vi "CTRE_Phoenix_MotorController_GetClosedLoopData.vi"(0 "PhoenixMotorControlDevRef":T1={"DeviceStatus"={"status"=FALSE, "code"=0, "source"=""}, "Type"=enum."PWM", "PWM"={"PWM Channel"=enum."Invalid", "DeadBand"={"Name"="", "maxPositivePwm"=0, "minPositivePwm"=0, "centerPwm"=0, "maxNegativePwm"=0, "minNegativePwm"=0, "angularRange"=0}}, "CAN"={"Device Number"=0, "SetOutput VI Ref"=variant(enum8{"Percent VBus", "Current", "Speed", "Position", "Voltage"} enum."Percent VBus"), "GetOutput VI Ref"=variant(refnum<k1> refnum), "Enable VI Ref"=variant(dbl 12.0), "Disable VI Ref"=variant(enum8{"Percent VBus", "Speed", "Position", "Slave", "Unchanged / Invalid", "Voltage Compensation", "Current", "Motion Profile"} enum."Percent VBus"), "Data"=variant}, "Invert"=FALSE, "DIO PWM"={"PWM \"Enable\" Channel"=enum."Invalid", "DIOChannel"=enum."Invalid", "PWM Rate"=0.0}}, 5 "pidLoopIdx":i32, 11 "error in":errorcluster) -> (3 "Closed-loop Target":i32, 4 "PhoenixMotorControlDevRef":T1={"DeviceStatus"={"status"=FALSE, "code"=0, "source"=""}, "Type"=enum."PWM", "PWM"={"PWM Channel"=enum."Invalid", "DeadBand"={"Name"="", "maxPositivePwm"=0, "minPositivePwm"=0, "centerPwm"=0, "maxNegativePwm"=0, "minNegativePwm"=0, "angularRange"=0}}, "CAN"={"Device Number"=0, "SetOutput VI Ref"=variant(enum8{"Percent VBus", "Current", "Speed", "Position", "Voltage"} enum."Percent VBus"), "GetOutput VI Ref"=variant(refnum<k1> refnum), "Enable VI Ref"=variant(dbl 12.0), "Disable VI Ref"=variant(enum8{"Percent VBus", "Speed", "Position", "Slave", "Unchanged / Invalid", "Voltage Compensation", "Current", "Motion Profile"} enum."Percent VBus"), "Data"=variant}, "Invert"=FALSE, "DIO PWM"={"PWM \"Enable\" Channel"=enum."Invalid", "DIOChannel"=enum."Invalid", "PWM Rate"=0.0}}, 6 "Closed-loop Error":i32, 8 "Error Derivative":dbl, 10 "Integral Accumulator":dbl, 15 "error out":errorcluster)   [LabVIEW 2017]
doc: "<b> pidLoopIdx </b> The selected PID object to retrieve information from. Select 0 for primary, 1 for secondary (cascaded) PID loop.\nReturns the closed-loop data of the motor controller, including:\n\nClosed-loop Target\nClosed-loop Error\nError Derivative\nIntegral Accumulator"
uses:
  <vilib>/Rock Robotics/WPI/MotorControl/WPI_MotorControlDeviceRef.ctl
  <vilib>/Rock Robotics/WPI/MotorControl/WPI_MotorControlType.ctl
  <vilib>/Rock Robotics/SystemInterfaces/DIO/FPGA_DIOPWMChannel.ctl
  <vilib>/Rock Robotics/WPI/PWM/WPI_PWMDeadband.ctl
  <vilib>/Rock Robotics/SystemInterfaces/DIO/FPGA_DIOChannel.ctl
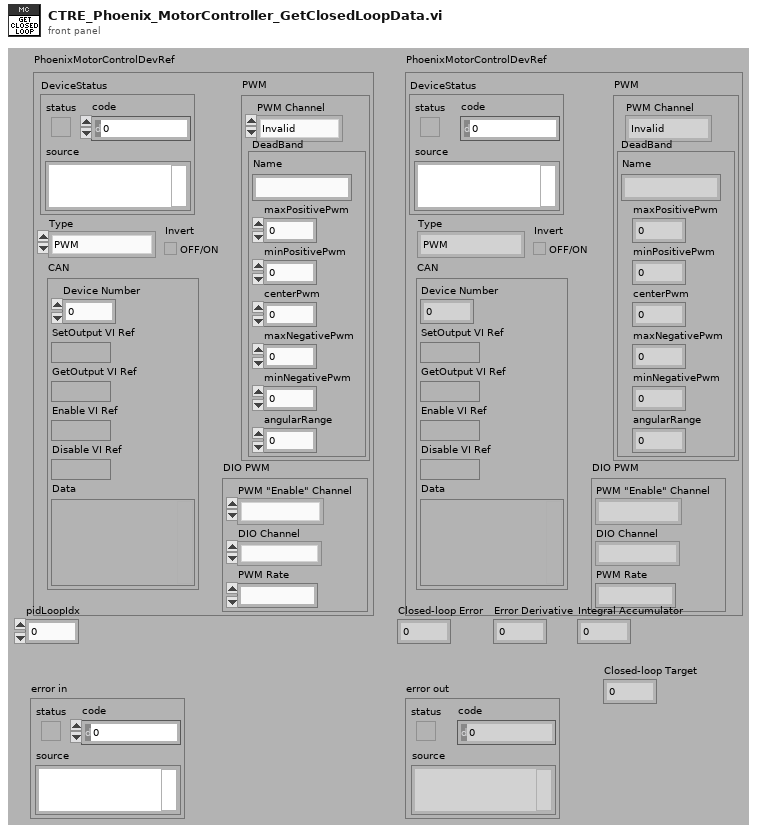
[diagram p1: front panel]
types:
  T1 = typedef "WPI_MotorControlDeviceRef.ctl" = cluster{"DeviceStatus":errorcluster, "Type":T2, "PWM":cluster{"PWM Channel":T3, "DeadBand":T4}, "CAN":cluster{"Device Number":u8, "SetOutput VI Ref":variant, "GetOutput VI Ref":variant, "Enable VI Ref":variant, "Disable VI Ref":variant, "Data":variant}, "Invert":bool, "DIO PWM":cluster{"PWM \"Enable\" Channel":T3, "DIOChannel":T5, "PWM Rate":dbl}}
  T2 = typedef "WPI_MotorControlType.ctl" = enum16{"PWM", "CAN", "DIO PWM"}
  T3 = typedef "FPGA_DIOPWMChannel.ctl" = enum8{"PWM 0", "PWM 1", "PWM 2", "PWM 3", "PWM 4", "PWM 5", "PWM 6", "PWM 7", "PWM 8", "PWM 9", "PWM MXP 0", "PWM MXP 1", "PWM MXP 2", "PWM MXP 3", "PWM MXP 4", "PWM MXP 5", "PWM MXP 6", "PWM MXP 7", "PWM MXP 8", "PWM MXP 9", "Invalid"}
  T4 = typedef "WPI_PWMDeadband.ctl" = cluster{"Name":string, "maxPositivePwm":i32, "minPositivePwm":i32, "centerPwm":i32, "maxNegativePwm":i32, "minNegativePwm":i32, "angularRange":u16}
  T5 = typedef "FPGA_DIOChannel.ctl" = enum8{"DIO 0", "DIO 1", "DIO 2", "DIO 3", "DIO 4", "DIO 5", "DIO 6", "DIO 7", "DIO 8", "DIO 9", "DIO MXP 0", "DIO MXP 1", "DIO MXP 2", "DIO MXP 3", "DIO MXP 4", "DIO MXP 5", "DIO MXP 6", "DIO MXP 7", "DIO MXP 8", "DIO MXP 9", "DIO MXP 10", "DIO MXP 11", "DIO MXP 12", "DIO MXP 13", "DIO MXP 14", "DIO MXP 15", "SPI Port CS1", "SPI Port CS2", "SPI Port CS3", "SPI Port MISO", "SPI Port MOSI", "Invalid"}
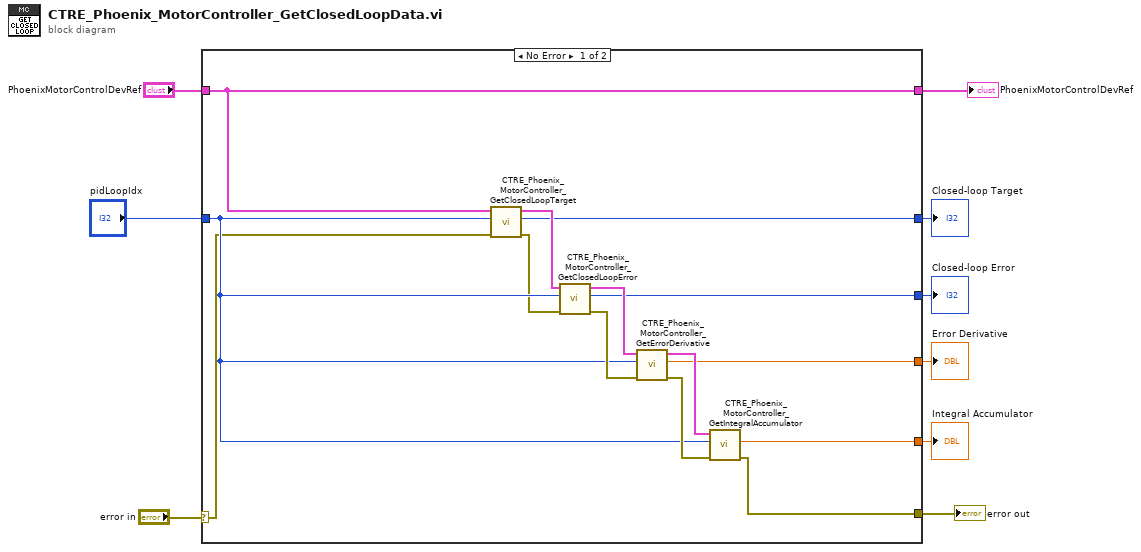
[diagram p0: block diagram]
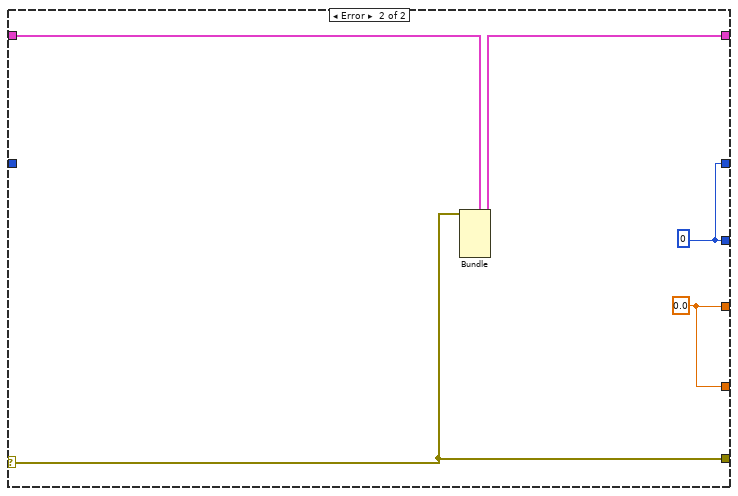
[diagram p2: hidden frame]
diagram:
  n1 = case shown="No Error" "error in" {
    selector: "error in" -> [w12 w27]
    tunnel: "PhoenixMotorControlDevRef" -> [w15 w28]
    tunnel: [w16 w27] -> w8
    tunnel: [w15 w26] -> w6
    tunnel: [w19 w24] -> w5
    tunnel: [w18 w25] -> w4
    tunnel: [w17 w25] -> w3
    tunnel: "pidLoopIdx" -> [w14 _]
    tunnel: [w10 w24] -> w1
    frame No Error {
      n2 = call "CTRE_Phoenix_MotorController_GetClosedLoopTarget.vi"("error in"=w12, "pidLoopIdx"=w14, "PhoenixMotorControlDevRef"=w15) -> ("error out"=w11:errorcluster, "Closed-loop Target"=w10:i32, "PhoenixMotorControlDevRef"=w13:T1)  [unwired: 6 in]
      n3 = call "CTRE_Phoenix_MotorController_GetClosedLoopError.vi"("error in"=w11, "pidLoopIdx"=w14, "PhoenixMotorControlDevRef"=w13) -> ("error out"=w21:errorcluster, "Closed-loop Error"=w19:i32, "PhoenixMotorControlDevRef"=w23:T1)  [unwired: 6 in]
      n4 = call "CTRE_Phoenix_MotorController_GetErrorDerivative.vi"("error in"=w21, "pidLoopIdx"=w14, "PhoenixMotorControlDevRef"=w23) -> ("error out"=w20:errorcluster, "Error Derivative"=w18:dbl, "PhoenixMotorControlDevRef"=w22:T1)  [unwired: 6 in]
      n5 = call "CTRE_Phoenix_MotorController_GetIntegralAccumulator.vi"("PhoenixMotorControlDevRef"=w22, "pidLoopIdx"=w14, "error in"=w20) -> ("Integral Accumulator"=w17:dbl, "error out"=w16:errorcluster)  [unwired: 5 in, 1 out]
    }
    frame Error {
      w24 = 0 ("Closed-loop Error")
      w25 = 0.0 ("Closed-loop Error")
      n6 = Bundle(cluster=w28, "DeviceStatus"=w27) -> (w26:T1)  [unwired: 5 in]
    }
  }
  "PhoenixMotorControlDevRef" <- w6
  "error out" <- w8
  "Closed-loop Error" <- w5
  "Error Derivative" <- w4
  "Integral Accumulator" <- w3
  "Closed-loop Target" <- w1
